vi "Aux TE Controllers Set SetPoints.vi"(6 "Set Point2":sgl, 8 "Error In":errorcluster, 9 "Set Point1":sgl, 11 "TE Serial Ports In":T1[](array[typedef]) {"XOFF Char" format="%.0x"; "XON Char" format="%.0x"; "flow control" items=["None"=0, "XON/XOFF"=1, "RTS/CTS"=2, "DTR/DSR"=4]; "stop bits" items=["1.0"=10, "1.5"=15, "2.0"=20]; "data bits" min=5 max=8 step=1; "baud rate" items=["75"=75, "110"=110, "134"=134, "150"=150, "300"=300, "600"=600, "1200"=1200, "1800"=1800, "2400"=2400, "4800"=4800, "7200"=7200, "9600"=9600, "14400"=14400, "19200"=19200, "28800"=28800, "38400"=38400, "56000"=56000, "57600"=57600, "115200"=115200, "128000"=128000, "230400"=230400]; "termination char" format="%.0x"}) -> (0 "Error Out":errorcluster, 2 "Error":bool, 3 "TE Serial Ports Out":T1[](array[typedef]) {"XOFF Char" format="%.0x"; "XON Char" format="%.0x"; "flow control" items=["None"=0, "XON/XOFF"=1, "RTS/CTS"=2, "DTR/DSR"=4]; "stop bits" items=["1.0"=10, "1.5"=15, "2.0"=20]; "data bits" min=5 max=8 step=1; "baud rate" items=["75"=75, "110"=110, "134"=134, "150"=150, "300"=300, "600"=600, "1200"=1200, "1800"=1800, "2400"=2400, "4800"=4800, "7200"=7200, "9600"=9600, "14400"=14400, "19200"=19200, "28800"=28800, "38400"=38400, "56000"=56000, "57600"=57600, "115200"=115200, "128000"=128000, "230400"=230400]; "termination char" format="%.0x"})   [LabVIEW 2016]
uses:
  Controls/Serial Visa Control.ctl
  Controls/SerialPortControl.ctl
panel:
  out "Data Read":string[](array[string])
  out "Loop active 2":bool
  out "Loop active":bool
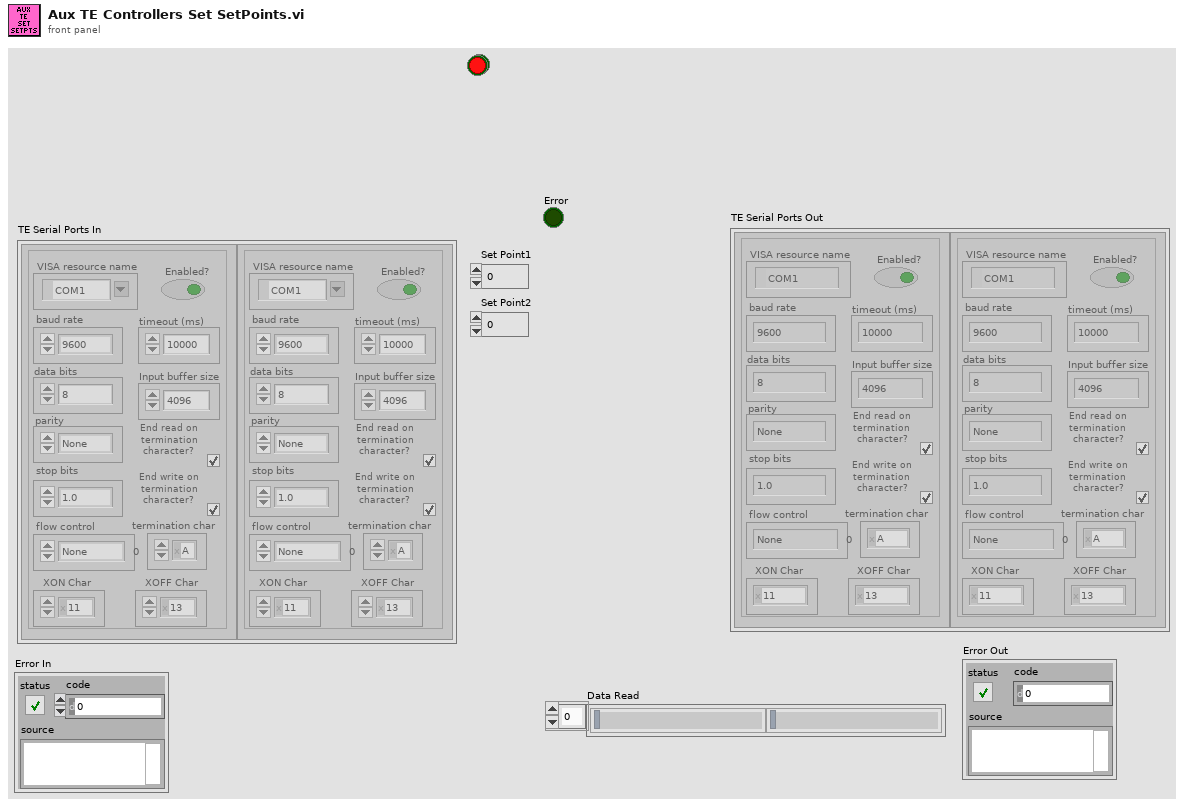
[diagram p1: front panel]
types:
  T1 = typedef "Serial Visa Control.ctl" = cluster{"termination char":u8, "End read on termination character?":bool, "Enabled?":bool, "VISA resource name":refnum<visa-resource-name>, "baud rate":u32, "data bits":u16, "parity":enum16{"None", "Odd", "Even", "Mark", "Space"}, "stop bits":u16, "flow control":u16, "timeout (ms)":u32, "Input buffer size":u32, "End write on termination character?":bool, "XON Char":u8, "XOFF Char":u8}
  T2 = typedef "SerialPortControl.ctl" = enum16{"Initialize", "Write Data", "Read Data", "Close Port"}
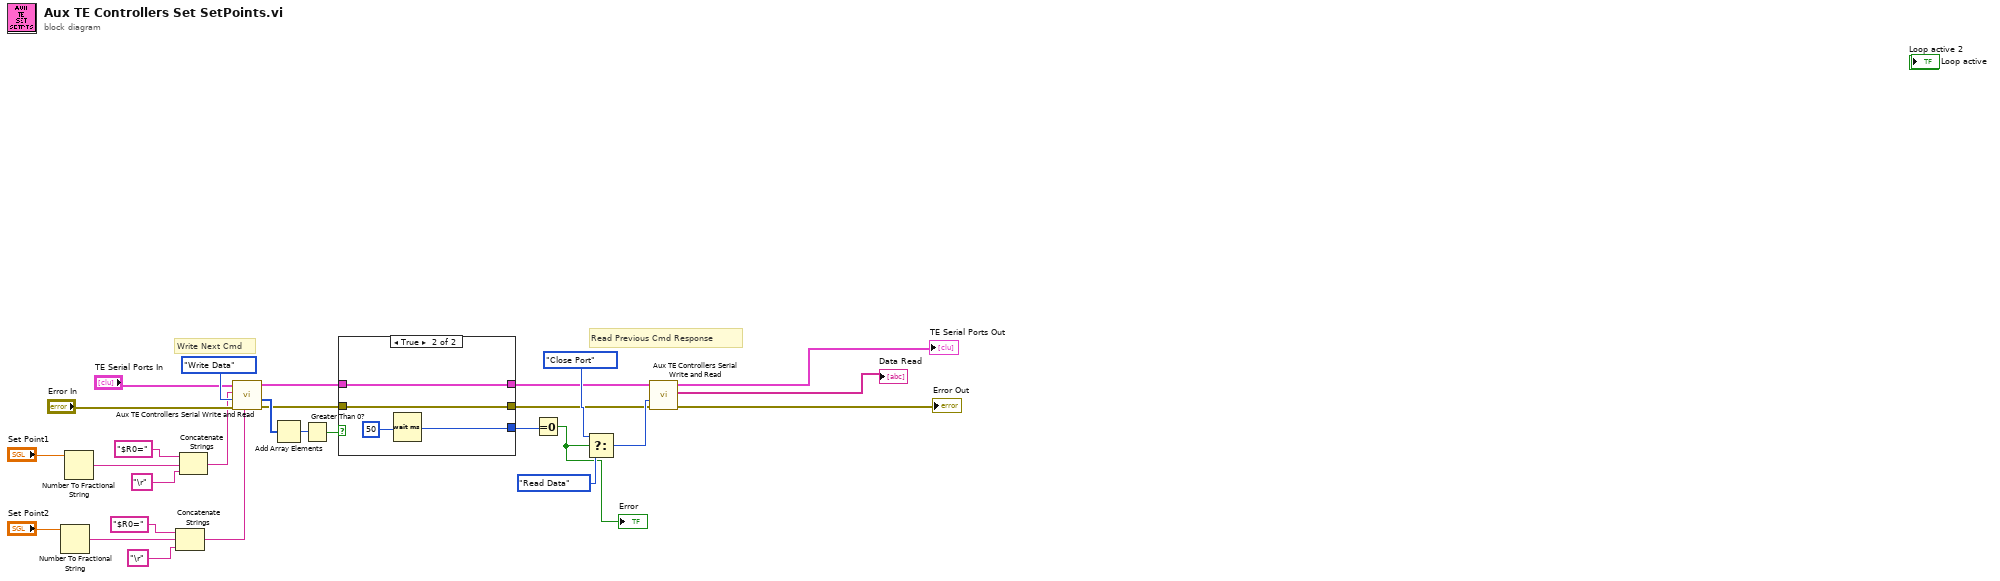
[diagram p0: block diagram]
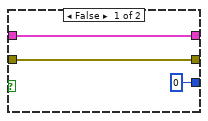
[diagram p2: hidden frame]
diagram:
  # "Read Previous Cmd Response"
  # "Write Next Cmd"
  n1 = Number To Fractional String(number="Set Point2") -> (F-format string=w27:string)  [unwired: 3 in]
  n2 = Number To Fractional String(number="Set Point1") -> (F-format string=w24:string)  [unwired: 3 in]
  n3 = Concatenate Strings("$R0=" ("string to write"), w27, "\r" ("string to write")) -> (w2:string)
  n4 = Concatenate Strings("$R0=" ("string to write"), w24, "\r" ("string to write")) -> (w3:string)
  n5 = call "Aux TE Controllers Serial Write and Read.vi"("second string"=w2, "error in"="Error In", "Action"=SerialPortControl."Write Data", "string to write"=w3, "TE Controller Serial Ports In"="TE Serial Ports In") -> ("Error Out"=w12:errorcluster, "#Bytes R/W"=w16:i16[], "TE Controller Serial Ports Out"=w10:T1[])  [unwired: 2 out]
  n6 = Add Array Elements(numeric array=w16) -> (sum=w14:i16)
  n7 = Greater Than 0?(x=w14) -> (x > 0?=w15:bool)
  n8 = case shown="True" w15 {
    tunnel: [w30 w35] -> w11
    tunnel: w10 -> [w30 w35]
    tunnel: [w31 w34] -> w13
    tunnel: w12 -> [w31 w34]
    tunnel: [u32 0 ("millisecond timer value") w32] -> w17
    frame False {
    }
    frame True {
      n9 = Wait (ms)(milliseconds to wait=i16 50 ("y")) -> (millisecond timer value=w32:u32)
    }
  }
  n10 = Equal To 0?(x=w17) -> (x = 0?=w1:bool)
  "Error" <- w1
  n11 = Select(t=SerialPortControl."Close Port" ("Action"), s=w1, f=SerialPortControl."Read Data" ("Action")) -> (s? t:f=w18:T2)
  n12 = call "Aux TE Controllers Serial Write and Read.vi"("error in"=w13, "Action"=w18, "TE Controller Serial Ports In"=w11) -> ("Error Out"=→"Error Out":errorcluster, "Data Read"=→"Data Read":string[], "TE Controller Serial Ports Out"=→"TE Serial Ports Out":T1[])  [unwired: 2 in, 2 out]
